vi "Create Resource (Bus).vi"(0 "reference fpga in":refnum<class "niUSRP Reference FPGA v1.lvclass">) -> (4 "reference fpga out":refnum<class "niUSRP Reference FPGA v1.lvclass">)   [LabVIEW 2025, in "niUSRP Reference FPGA v1.lvclass"]
uses:
  niUSRP Reference FPGA v1.lvclass
  niUSRP Reference FPGA v1.lvclass/niUSRP Reference FPGA v1.ctl
  <instrlib>/_niInstr/FIFO Register Bus/v1/FPGA/niInstr FIFO Register Bus v1 FPGA.lvclass
  C:/Program Files/NI/LVAddons/niidl/1/instr.lib/_niInstr/Instruction Framework/v1/FPGA/Interfaces/Instruction Producer/Instruction Producer.lvclass
  <instrlib>/_niInstr/Instruction Framework/v1/FPGA/Top Level Bus/Register Configuration/Register Configuration.lvclass
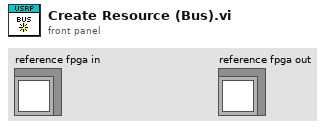
[diagram p1: front panel]
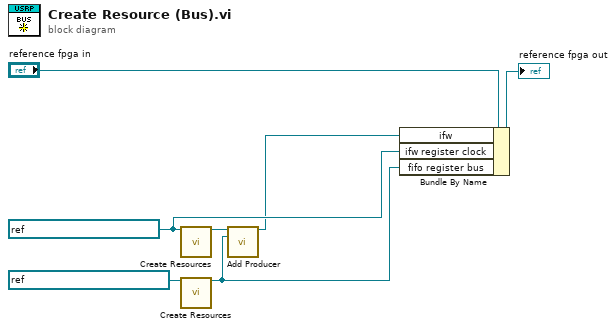
[diagram p0: block diagram]
diagram:
  w2 = refnum<k21> "40 MHz Onboard Clock" ("register clock")
  n1 = call <instrlib>:"Create Resources.vi"("register clock"=w2) -> ("register configuration"=w6:refnum<class "Register Configuration.lvclass">)  [unwired: 14 in]
  n2 = call <instrlib>:"Create Resources.vi"("instruction fifo"=refnum<k21> "reg.host instruction fifo 0") -> ("fifo register bus"=w3:refnum<class "niInstr FIFO Register Bus v1 FPGA.lvclass">)  [unwired: 14 in]
  n3 = call-dynamic "Add Producer.vi"("register configuration in"=w6, "instruction producer"=w3) -> ("register configuration out"=w1:refnum<class "Register Configuration.lvclass">)  [unwired: 13 in]
  n4 = Bundle By Name(cluster="reference fpga in", "ifw"=w1, "ifw register clock"=w2, "fifo register bus"=w3) -> (→"reference fpga out":refnum<class "niUSRP Reference FPGA v1.lvclass">)
